vi "Multiple Instances.vi"() -> ()   [LabVIEW 2024]
uses:
  <vilib>/sklein/WebView2/Webview2 Control/WebView2 Control.xctl
panel:
  out "WebView2 Control 1":string(xcontrol)
  out "WebView2 Control 2":string(xcontrol)
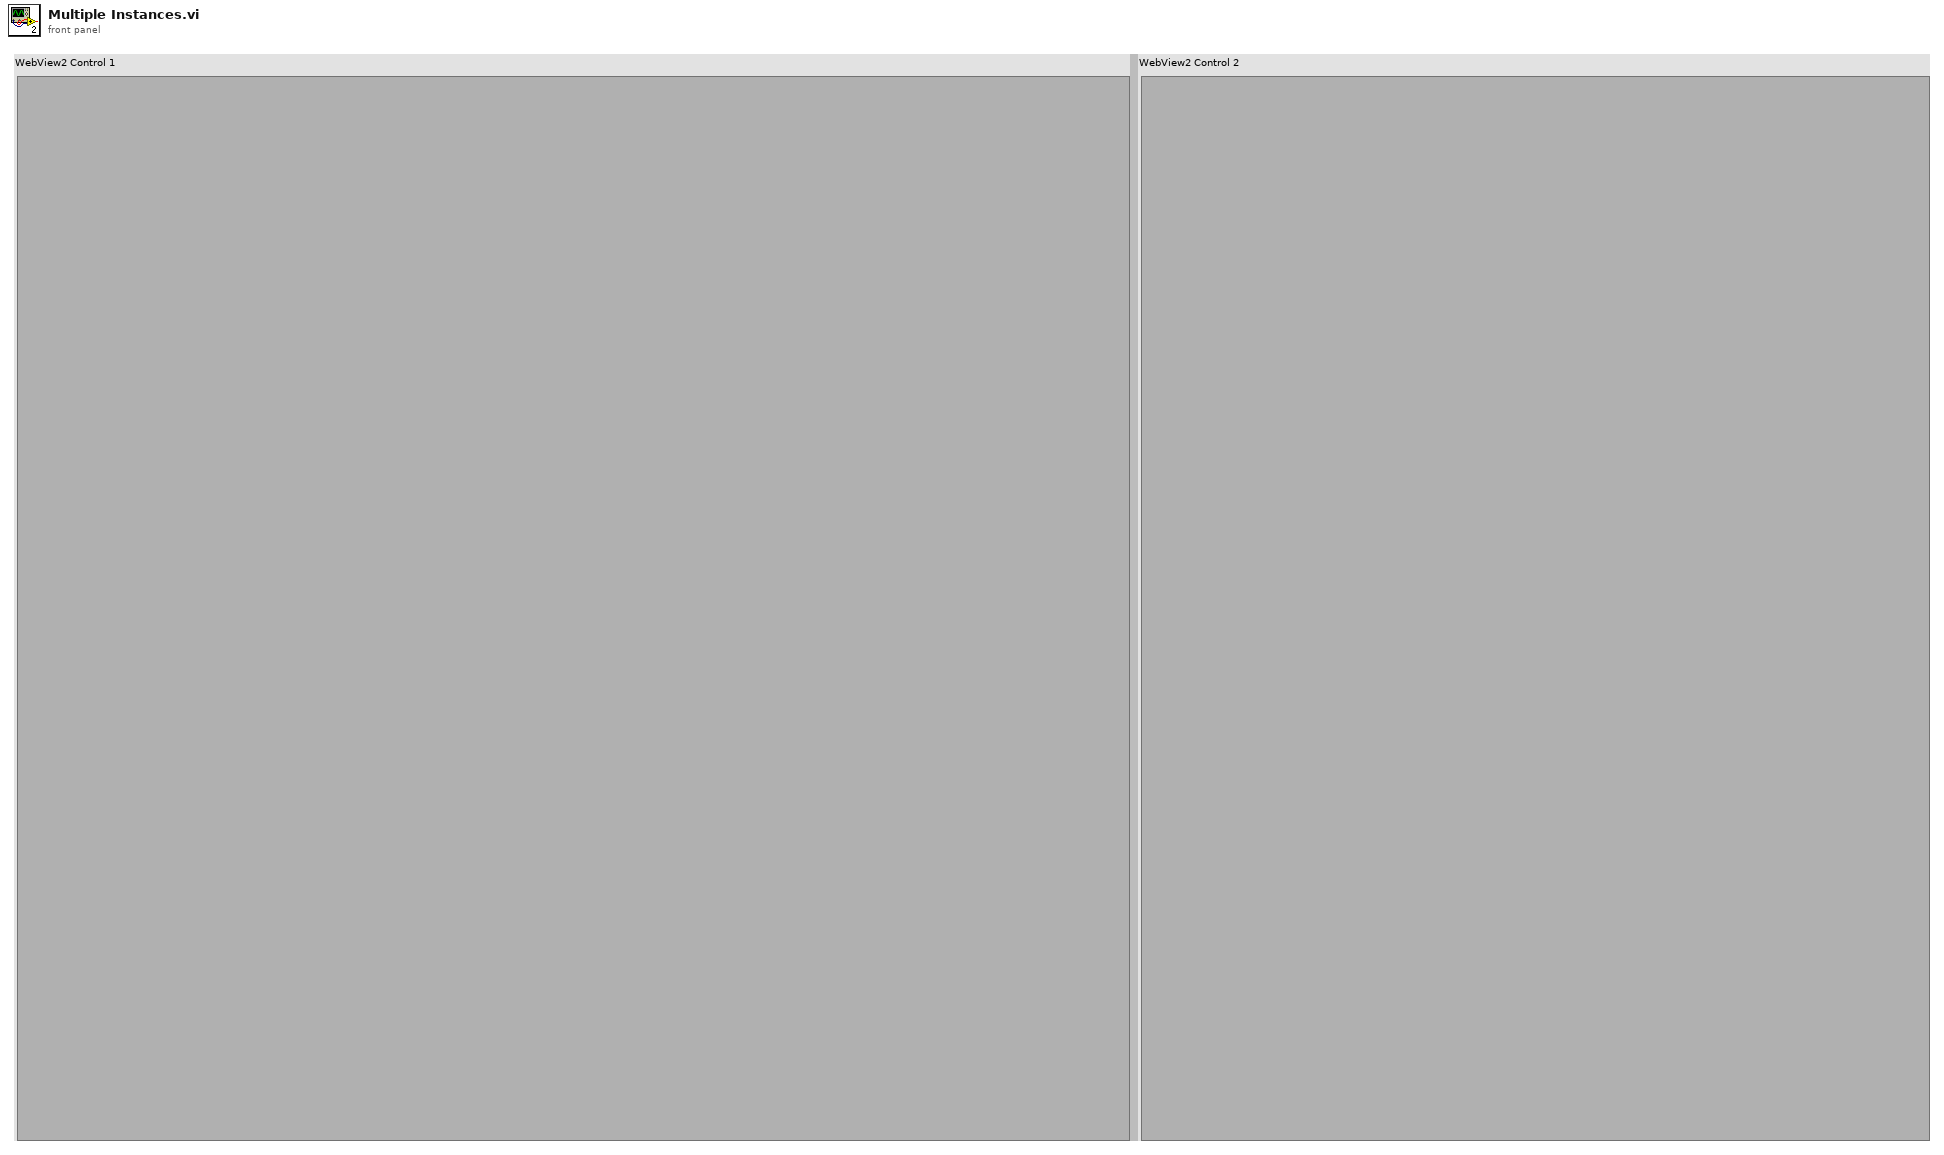
[diagram p1: front panel]
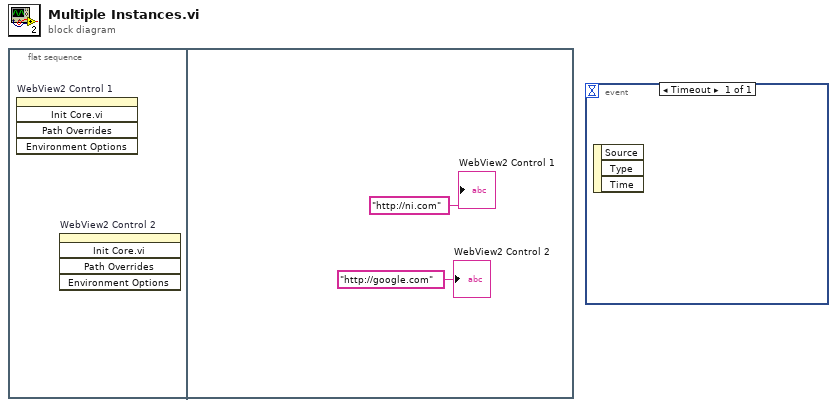
[diagram p0: block diagram]
diagram:
  n1 = flat-sequence {
    frame #0 {
      n2 = invoke on="WebView2 Control 1" class="WebView2 Control (strict)" method="Init Core.vi"() -> ()  [unwired: 5 in, 5 out]
      n3 = invoke on="WebView2 Control 2" class="WebView2 Control (strict)" method="Init Core.vi"() -> ()  [unwired: 5 in, 5 out]
    }
    frame #1 {
      "WebView2 Control 1" <- "http://ni.com" ("WebView2 Control")
      "WebView2 Control 2" <- "http://google.com" ("WebView2 Control 2")
    }
  }
  n4 = event shown="[0] Timeout" {
    selector: _ -> [_]
    dyn-events: _ -> [_]
    timeout: _ -> [_]
    event Timeout {
      n5 = event-data() -> ()  [unwired: 1 in, 3 out]
    }
  }
